vi "Array to String.vi"(11 "Array":string[](array[string])) -> (3 "String":string)   [LabVIEW 2014]
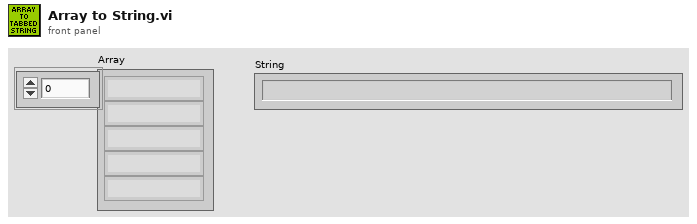
[diagram p1: front panel]
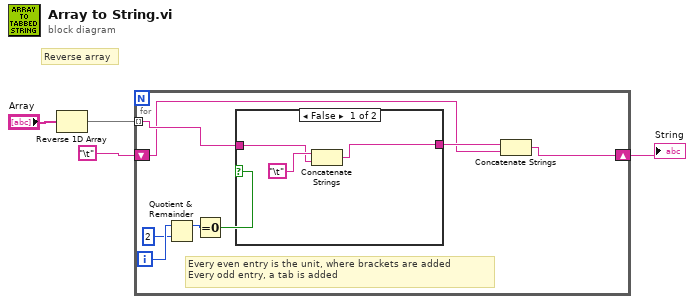
[diagram p0: block diagram]
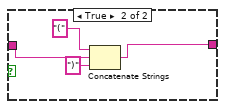
[diagram p2: hidden frame]
diagram:
  # "Reverse array"
  n1 = Reverse 1D Array(array="Array") -> (reversed array=w3:string[])
  n2 = for {
    tunnel: w3 -> [w8] mode=indexing
    shift-right: [w7] -> w1
    shift-left: "\t" -> [w5]
    i -> [w12]
    # "Every even entry is the unit, where brackets are added\nEvery odd entry, a tab is added"
    n3 = Quotient & Remainder(x=w12, y=2) -> (x-y*floor(x/y)=w10:i32)  [unwired: 1 out]
    n4 = Equal To 0?(x=w10) -> (x = 0?=w9:bool)
    n5 = case shown="False" w9 {
      tunnel: [w15 w18] -> w6
      tunnel: w8 -> [w13 w17]
      frame False {
        n6 = Concatenate Strings "Concatenate Strings"("\t", w13) -> (w15:string)
      }
      frame True {
        n7 = Concatenate Strings "Concatenate Strings"("(" ("string"), w17, ")" ("string")) -> (w18:string)
      }
    }
    n8 = Concatenate Strings "Concatenate Strings"(w6, w5) -> (w7:string)
  }
  "String" <- w1
